vi "LVFunction_Imop_Compute_Pupil_HasHoles.vi"(0 "Pupil.lvclass":refnum<class "Pupil.lvclass">, 11 "error in":errorcluster) -> (4 "Pupil.lvclass":refnum<class "Pupil.lvclass">, 6 "has_holes":bool, 15 "error out":errorcluster)   [LabVIEW 2018]
doc: "Compute the geometric parameters of the Legendre pupil from a cPupil input.\n\n--------------------------------------------------------------------------------\n\nPupilIn\n cPupil object.\n\nPupilOut\n cPupil object.\n\ncenter\n center coordinates.\n\nsize\n dimensions (width, height) of the square pupil detected\n\nErrorIn\n Error\nErrorOut\n Error"
uses:
  Classes/Pupil/Pupil.lvclass
  Classes/Pupil/LVClass_Pupil Read Pupil.vi
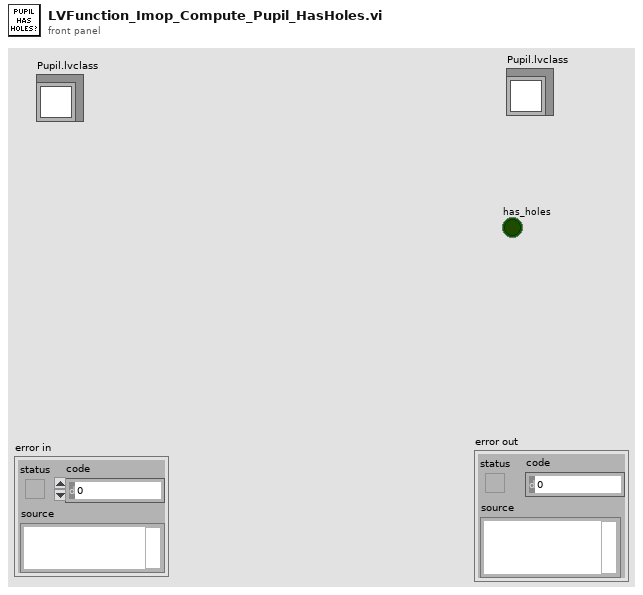
[diagram p1: front panel]
types:
  T1 = typedef "ClassID.ctl" = i64
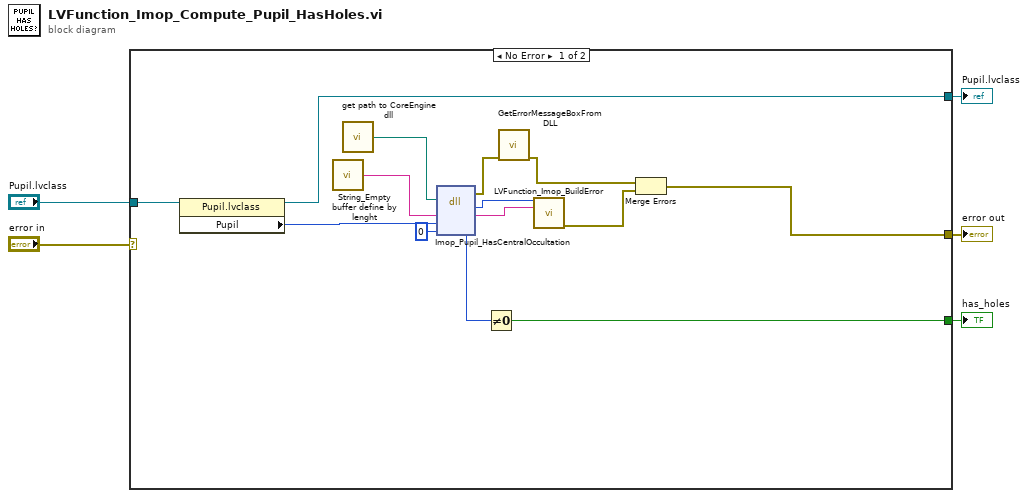
[diagram p0: block diagram]
diagram:
  n1 = case shown="No Error" "error in" {
    selector: "error in" -> [_ w21]
    tunnel: "Pupil.lvclass" -> [w7 w20]
    tunnel: [w18 w21] -> w3
    tunnel: [w6 w20] -> w2
    tunnel: [w8 _] -> w1
    frame No Error {
      n2 = property class="Pupil.lvclass"(reference=w7) -> (reference out=w6:refnum<class "Pupil.lvclass">, "Pupil"=w19:T1)  [unwired: 1 in, 1 out]
      n3 = call "String_Empty buffer define by lenght.vi"() -> ("Empty buffer"=w17:string)  [unwired: 1 in]
      n4 = call "get path to CoreEngine dll.vi"() -> ("path to wavekit library"=w14:path)  [unwired: 14 in, 1 out]
      n5 = dll-call lib="D:/FLE/0.Code/CoreEngine4_Suite/LV2011_interface/DLLs/c_interface_vc100.dll" fn="Imop_Pupil_HasCentralOccultation"(path in=w14, "message"=w17, "Pupil"=w19, "has_holes"=u8 0 ("center")) -> (error out=w13:errorcluster, "return type"=w15:i32, "message"=w16:string, "has_holes"=w9:u8)  [unwired: 3 in, 1 out]
      n6 = Not Equal To 0?(x=w9) -> (x != 0?=w8:bool)
      n7 = call "GetErrorMessageBoxFromDLL.vi"("error IN"=w13) -> ("error OUT"=w12:errorcluster)  [unwired: 10 in]
      n8 = call "LVFunction_Imop_BuildError.vi"("code"=w15, "String to Prepend to source (\"\")"=w16) -> ("error out"=w11:errorcluster)  [unwired: 13 in]
      n9 = Merge Errors(w12, w11) -> (w18:errorcluster)
    }
    frame Error {
    }
  }
  "error out" <- w3
  "Pupil.lvclass" <- w2
  "has_holes" <- w1
